vi "analog dynamic data.vi"() -> ()   [LabVIEW 2018]
panel:
  in  "stop":bool
  out "Meter":dbl(knob) scale=-10.0..10.0
  in  "Slide":dbl(slide) scale=-10.0..10.0
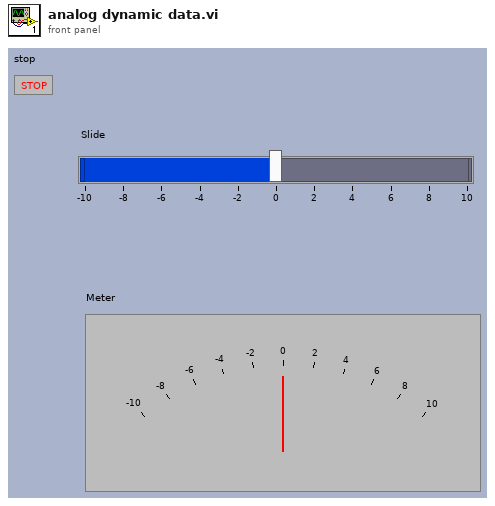
[diagram p1: front panel]
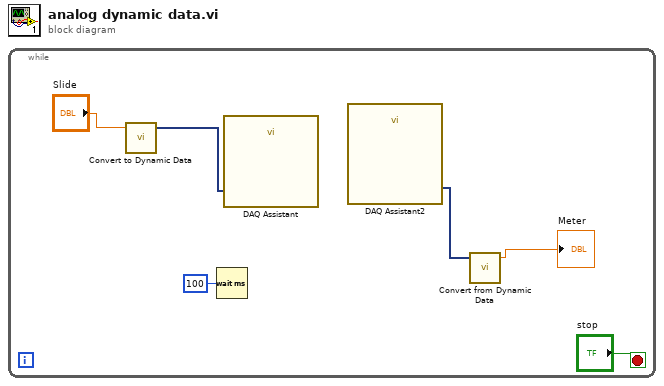
[diagram p0: block diagram]
diagram:
  n1 = while {
    stop <- "stop" stop-if-true
    n2 = call "Convert to Dynamic Data"("Double"="Slide") -> ("Dynamic Data Type"=w5:dynamicdata)  [unwired: 3 in]
    n3 = Wait (ms)(milliseconds to wait=u32 100) -> ()  [unwired: 1 out]
    n4 = call "DAQ Assistant"("data"=w5) -> ()  [unwired: 17 in, 2 out]
    n5 = call "DAQ Assistant2"() -> ("data"=w4:dynamicdata)  [unwired: 17 in, 2 out]
    n6 = call "Convert from Dynamic Data"("Dynamic Data Type"=w4) -> ("Scalar"=→"Meter":dbl)  [unwired: 3 in]
  }
